vi "getImageValueStimulus.vi"(8 "error in (no error)":errorcluster, 11 "Stimulus in":refnum<class "Stimulus.lvclass">) -> (0 "error out":errorcluster, 2 "Pixel Value (Float)":sgl format="%.2f", 3 "Stimulus out":refnum<class "Stimulus.lvclass">)   [LabVIEW 2014, in "Stimulus.lvclass"]
uses:
  Stimulus.lvclass
  Stimulus.lvclass/Stimulus.ctl
  <vilib>/vision/NI_Vision_Development_Module.lvlib
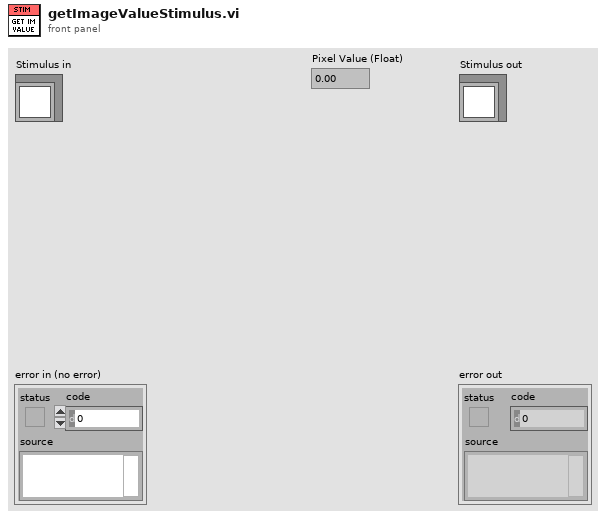
[diagram p1: front panel]
types:
  T1 = typedef "IMAQ Image.ctl" = refnum<image>
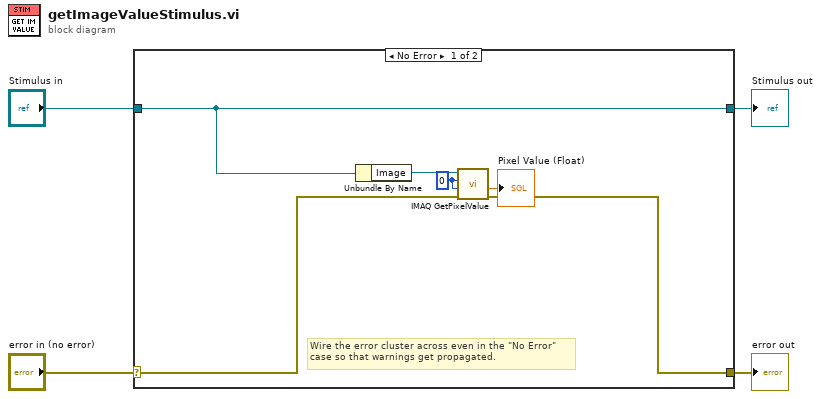
[diagram p0: block diagram]
diagram:
  n1 = case shown="No Error" "error in (no error)" {
    selector: "error in (no error)" -> [w8 w12]
    tunnel: [w7 w12] -> w3
    tunnel: [w5 w11] -> w1
    tunnel: "Stimulus in" -> [w5 w11]
    frame No Error {
      w9 = 0 ("X Coordinate")
      # "Wire the error cluster across even in the \"No Error\"\ncase so that warnings get propagated."
      n2 = Unbundle By Name(w5) -> ("Image"=w10:T1)
      n3 = call "IMAQ GetPixelValue"("Image"=w10, "X Coordinate"=w9, "Y Coordinate"=w9, "error in (no error)"=w8) -> ("Pixel Value (Float)"=→"Pixel Value (Float)":sgl, "error out"=w7:errorcluster)  [unwired: 2 in, 3 out]
    }
    frame Error {
    }
  }
  "error out" <- w3
  "Stimulus out" <- w1
